vi "LCR_Main.vi"() -> ()   [LabVIEW 2021]
uses:
  Sources/Plotting-Axis.ctl
  GEN_States.ctl
  Sources/Config_Cluster.ctl
  Sources/Mode_Enum.ctl
  Sources/Data_Cluster.ctl
  Sources/Measurement_Cluster.ctl
  1375486a-d526-4950-a4e9-ede105372d37.vi
  <vilib>/Utility/config.llb/NI_LVConfig.lvlib
panel:
  in  "Control Tab":enum32{"LCR Operation", "Configs"}(tab)
  out "Magnetic Field":dbl
  out "Temperature":dbl
  in  "RefreshM_Button":bool
  in  "Operation Mode":enum32{"Item 0", "Item 1", "Radio Selection 3"}(radio)
  out "Time Stamp":timestamp format="%<%H:%M:%S>T"
  out "Secondary":dbl format="%#_6p"
  out "Primary":dbl format="%#_6p"
  in  "SaveProfile_Button":bool
  in  "Send_Button":bool
  in  "LoadProfile_Button":bool
  in  "Measurement Profile":path
  in  "Tab Control":T1(tab)
  in  "Auto Range (T: Enable)":bool=TRUE
  in  "Circuit Type (2: Auto)":u16(ring)=2 items=["Series", "Parallel", "Auto"]
  in  "Operation Mode (0: Auto)":u16(ring) items=["Auto", "L+Q", "L+R", "C+D", "C+R", "R+Q", "Z+Theta", "Y+Theta", "R+X", "G+B", "N+Theta", "M"]
  in  "Manual Range (1:Range 1 and 25 Ohms)":u8(ring)=1 items=["Range 1 and 25 Ohms"=1, "Range 2 and 25 Ohms"=2, "Range 3 and 400 Ohms"=3, "Range 4 and 6.4 kOhms"=4, "Range 5 and 100kOhms"=5, "Range 6 and 100kOhms"=6]
  in  "Bias Source (OFF)":u8(ring) items=["Off", "Internal", "External"]
  in  "Bias Level (0)":dbl
  in  "Bias Type (Voltage)":u8(ring) items=["Voltage", "Current"]
  in  "Averaging (0: Off)":u16(ring) items=["Off", "Normal", "Averaging"]
  in  "Averaging Number (2)":i32=2 min=2 max=99
  in  "Rate (0: Fast)":u16(ring) items=["Fast", "Medium", "Slow"]
  in  "Time (100ms)":i32=100 min=1 max=999
  in  "Frequency (1kHz)":dbl=1000.0 min=20.0 max=200000.0
  in  "Measuring Voltage (1V)":dbl=1.0 min=0.05 max=1.5 step=0.01
  in  "Trigger Mode (0: Continuous)":u16(ring) items=["Continuous", "Manual", "External"]
  in  "Logfile Prefix":string
  in  "Logging Path":path
  in  "Measure rate (1/s)":i32
  in  "SaveConfig_Button":bool
  in  "Default Measurement Profile":path
  in  "Retry_Button":bool
  in  "Restart on Load":bool
  in  "Config Path (Blank is default)":path
  in  "LCR VISA COM":refnum<visa-resource-name>
  in  "Max Elements":i32=5000
  in  "Global Temp VAR":refnum<k21>
  in  "Global Mag VAR":refnum<k21>
  in  "Display Tab":enum32{"Program Monitor", "Test Plot"}(tab)
  out "Status":string
  out "B Lag":dbl
  out "T Lag":dbl
  out "Test Graph":cluster{"X":dbl, "Y":dbl}[](graph)
  in  "Y-Axis":T2
  in  "X-Axis":T2
  in  "Exit_Button":bool
  # "R&S HM8118 Settings"
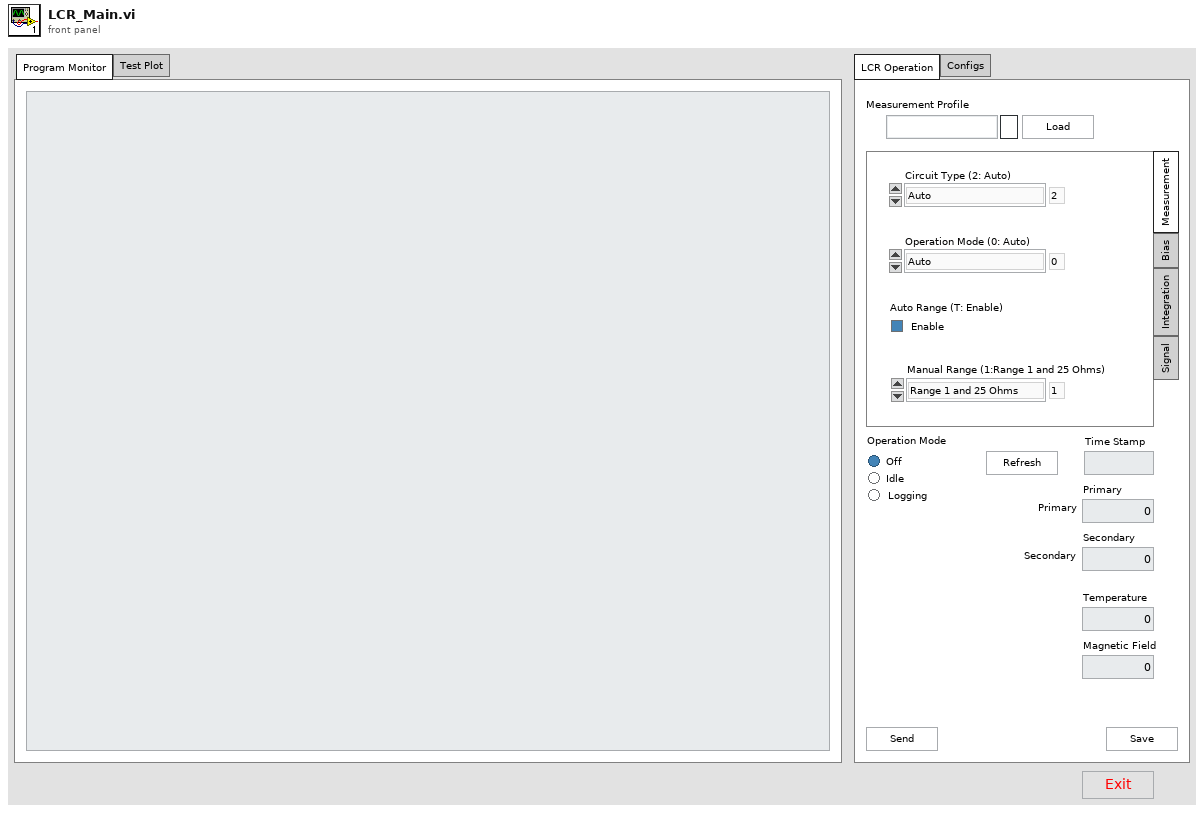
[diagram p1: front panel]
types:
  T1 = enum32{"Measurement", "Bias", "Integration", "Signal"}
  T2 = typedef "Plotting-Axis.ctl" = enum16{"Time", "Temperature", "MagneticField", "Primary", "Secondary"}
  T3 = typedef "GEN_States.ctl" = enum16{"UpdatePlots", "RefreshMUnits", "ChangeOperation", "Read/WriteAll", "RetryComs", "SendProfile", "InitGUI", "RefreshGUI", "ComsFail", "LoadProfile", "SaveProfile", "SaveConfig", "Idle", "ProgInit"}
  T4 = typedef "Data_Cluster.ctl" = cluster{"Value":dbl, "GUI Data Cluster":cluster{"Bias":cluster{"Bias Type (Voltage) 2":refnum<vi>, "Bias Level (0) 2":refnum<vi>, "Bias Source (OFF) 2":refnum<vi>}, "Measurement":cluster{"Auto Range (T: Enable) 2":refnum<vi>, "Manual Range (1:Range 1 and 25 Ohms) 2":refnum<vi>, "Operation Mode (0: Auto) 2":refnum<vi>, "Circuit Type (2: Auto) 2":refnum<vi>}, "Integration":cluster{"Rate (0: Fast) 2":refnum<vi>, "Time (100ms) 2":refnum<vi>, "Averaging (0: Off) 2":refnum<vi>, "Averaging Number (2) 2":refnum<vi>}, "Signal":cluster{"Trigger Mode (0: Continuous) 2":refnum<vi>, "Frequency (1kHz) 2":refnum<vi>, "Measuring Voltage (1V) 2":refnum<vi>}}, "Timing":cluster{"Last Operation":dbl}, "Measurements":T5[]}
  T5 = typedef "Measurement_Cluster.ctl" = cluster{"Time Stamp":timestamp, "Primary":dbl, "Secondary":dbl, "Temperature":dbl, "MagneticField":dbl}
  T6 = typedef "Config_Cluster.ctl" = cluster{"General":cluster{"Config.ini":path, "Default Logging Path":path}, "Hardware":cluster{"LCR VISA COM":refnum<visa-resource-name>, "Measure Rate (1/s)":i32, "Reset on Load?":bool, "Measure Profile":path, "Global T VAR":refnum<k21>, "Global B VAR":refnum<k21>}, "HM8118 Current Profile":cluster{"Bias Profile":cluster{" Bias Source (OFF)":u8, " Bias Type (Voltage)":u8, "Bias Level (0)":dbl}, "Measurement Profile":cluster{"Operation Mode (0: Auto)":u16, "Circuit Type (2: Auto)":u16, "Manual Range (1:Range 1 and 25 Ohms)":u8, "Auto Range (T: Enable)":bool}, "Signal Profile":cluster{"Frequency (1kHz)":dbl, "Measuring Voltage (1V)":dbl}, "Integration Profile":cluster{"Averaging (0: Off)":u16, "Averaging Number (2)":i32, "Time (100ms)":i32, "Rate (0: Fast)":u16}, "Trigger Profile":cluster{"Trigger Mode (0: Continuous)":u16}}, "HM8118 New Profile":cluster{"Bias Profile":cluster{" Bias Source (OFF)":u8, " Bias Type (Voltage)":u8, "Bias Level (0)":dbl}, "Measurement Profile":cluster{"Operation Mode (0: Auto)":u16, "Circuit Type (2: Auto)":u16, "Manual Range (1:Range 1 and 25 Ohms)":u8, "Auto Range (T: Enable)":bool}, "Signal Profile":cluster{"Frequency (1kHz)":dbl, "Measuring Voltage (1V)":dbl}, "Integration Profile":cluster{"Averaging (0: Off)":u16, "Averaging Number (2)":i32, "Time (100ms)":i32, "Rate (0: Fast)":u16}, "Trigger Profile":cluster{"Trigger Mode (0: Continuous)":u16}}, "Operation":cluster{"Operation Mode":T7, "Status":string}}
  T7 = typedef "Mode_Enum.ctl" = enum16{"Logging", "Idle-Off", "Idle"}
  T8 = enum8{"Enabled", "Disabled", "Disabled and Grayed Out"}
  T9 = typedef "NI_LVConfig.lvlib/Config Data RefNum.ctl" = refnum<k1>
  T10 = cluster{"Logging Path":path, "LCR VISA COM":refnum<visa-resource-name>, "Restart on Load":bool, "Default Measurement Profile":path, "Measure rate (1/s)":i32}
  T11 = cluster{"Primary Measurement":dbl, "Secondary Measurement":dbl, "T Var":dbl, "B Var":dbl}
  T12 = typedef "UnitEnum.ctl" = enum16{"L", "R", "C", "Z", "X", "Q", "Theta", "Y", "N", "M", "G", "B", "D"}
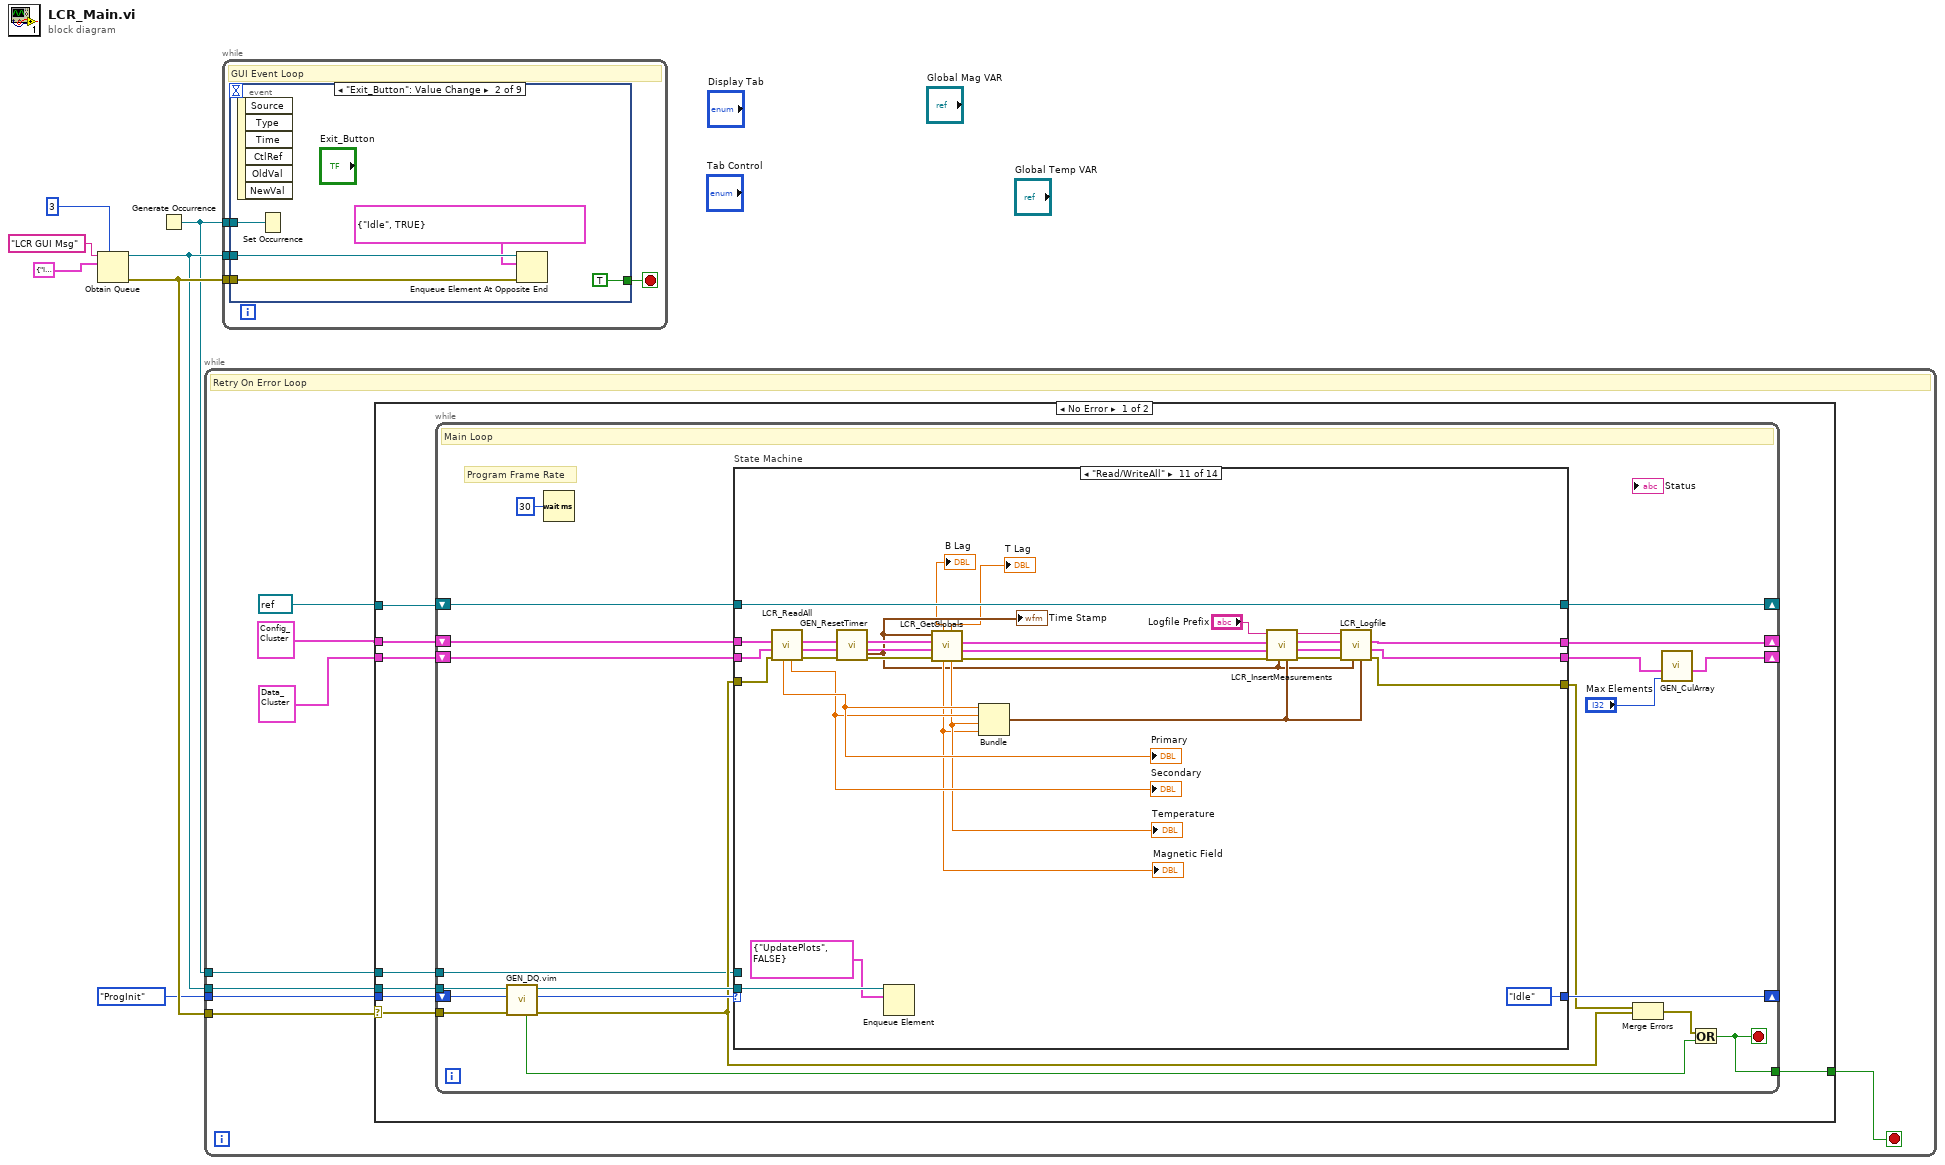
[diagram p0: block diagram]
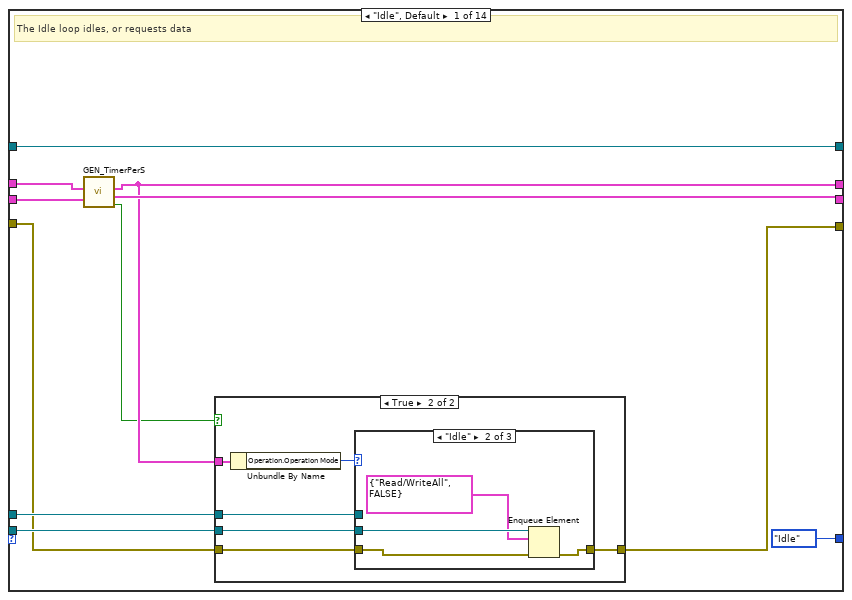
[diagram p2: hidden frame]
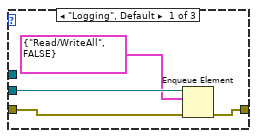
[diagram p4: hidden frame]
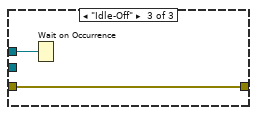
[diagram p5: hidden frame]
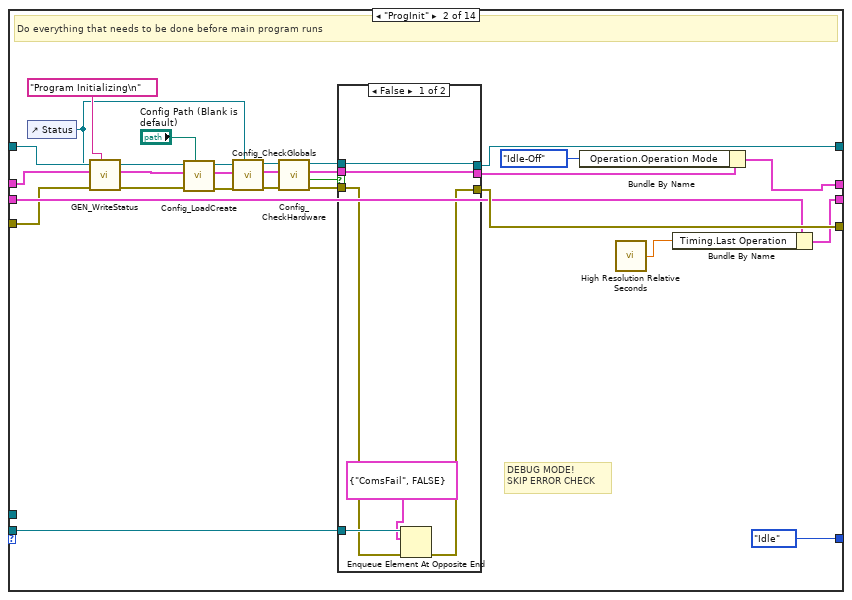
[diagram p6: hidden frame]
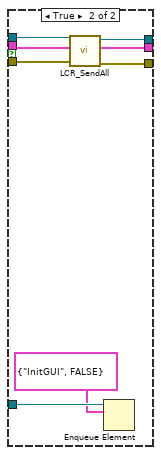
[diagram p7: hidden frame]
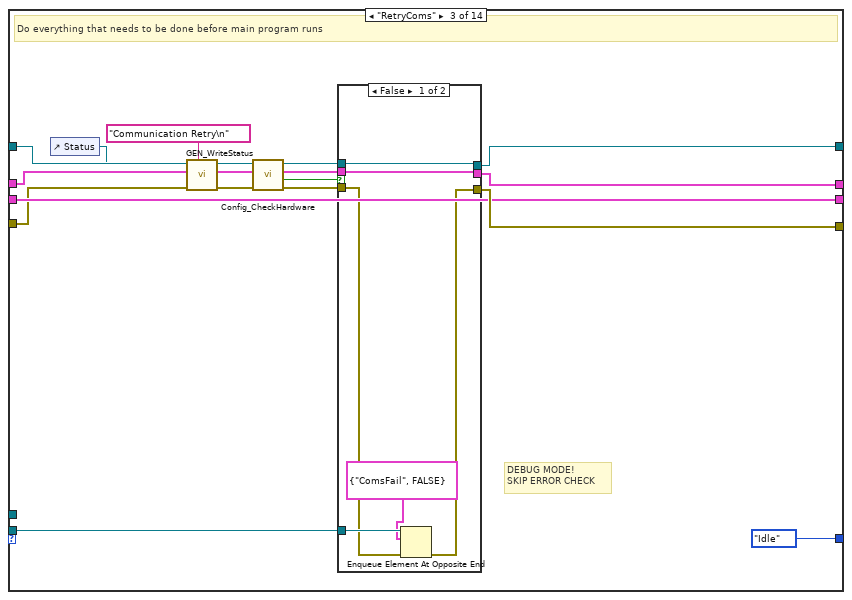
[diagram p8: hidden frame]
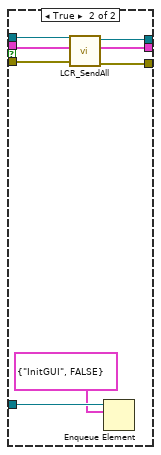
[diagram p9: hidden frame]
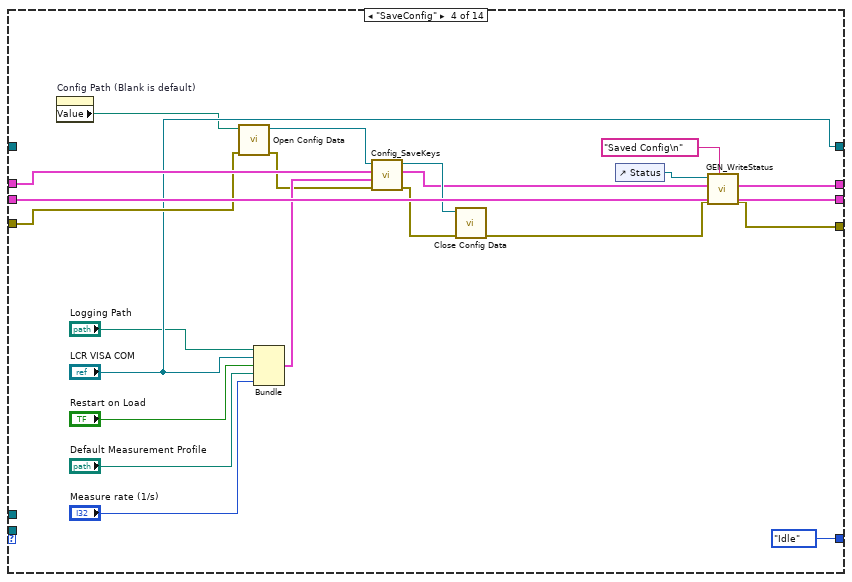
[diagram p10: hidden frame]
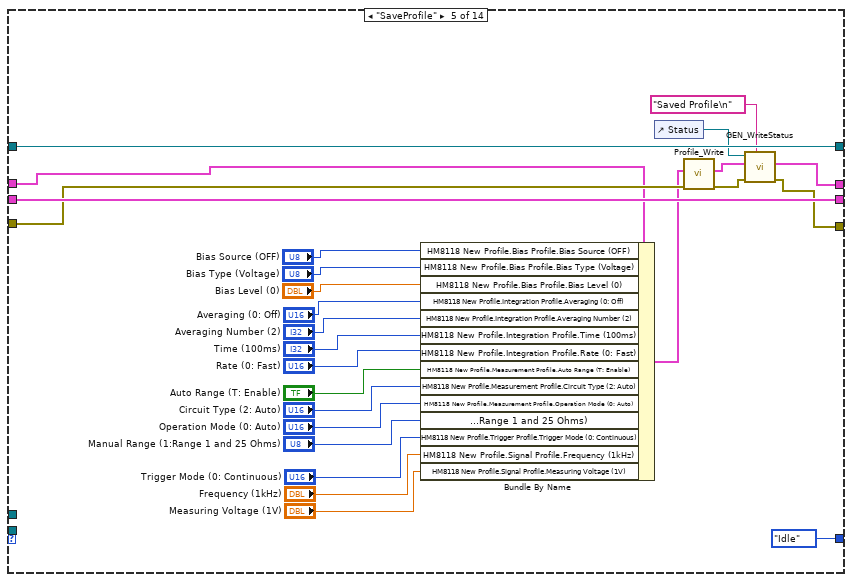
[diagram p11: hidden frame]
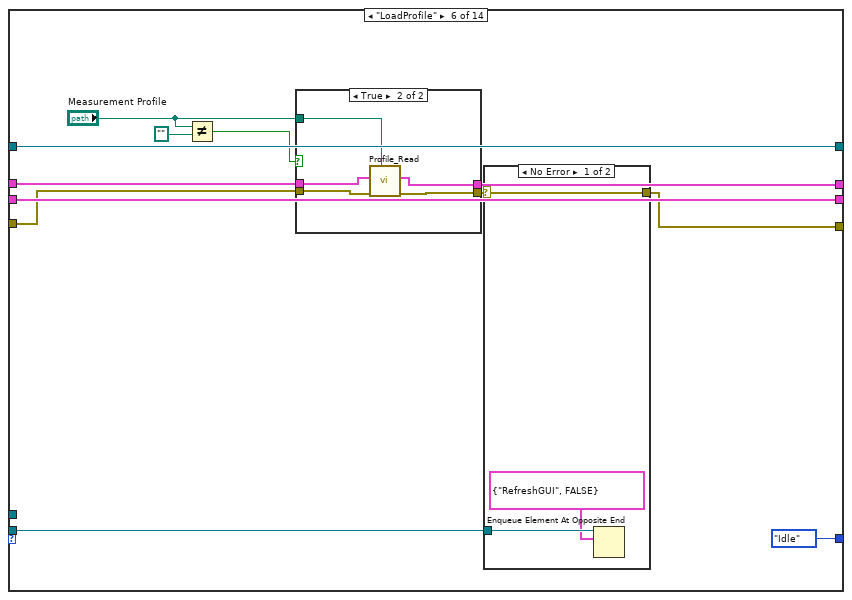
[diagram p12: hidden frame]
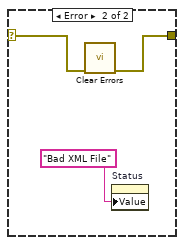
[diagram p13: hidden frame]
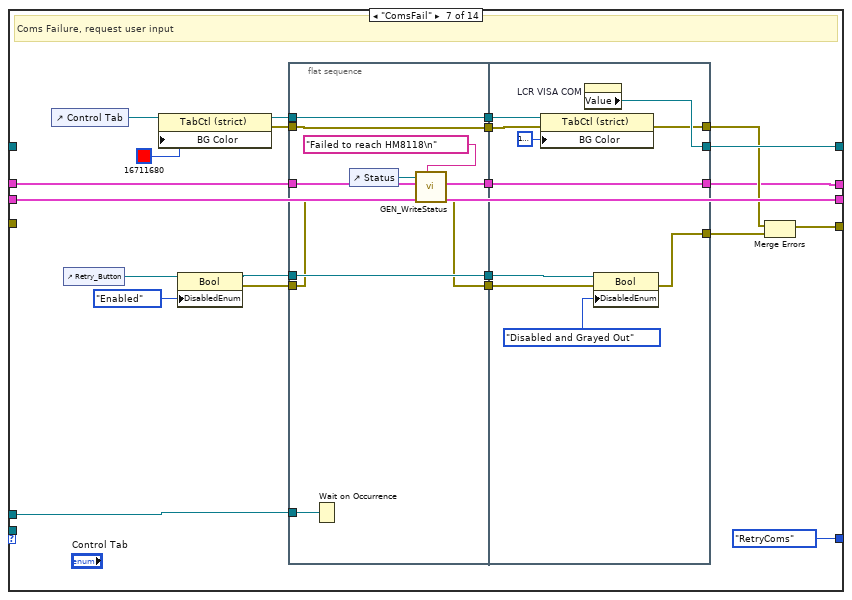
[diagram p15: hidden frame]
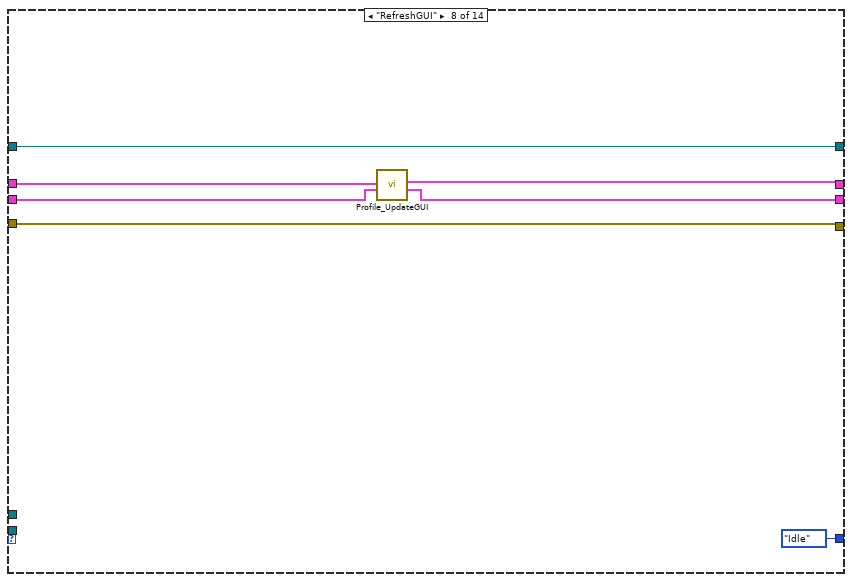
[diagram p16: hidden frame]
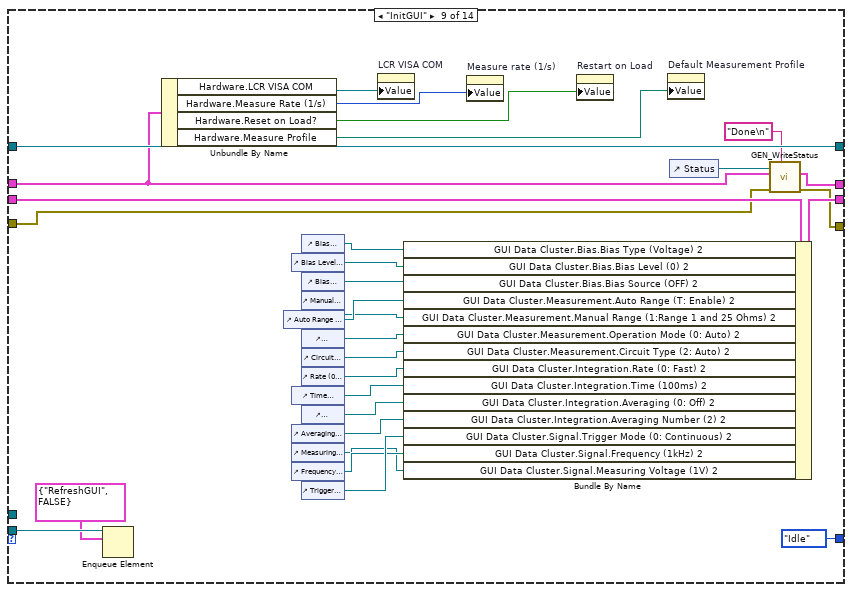
[diagram p17: hidden frame]
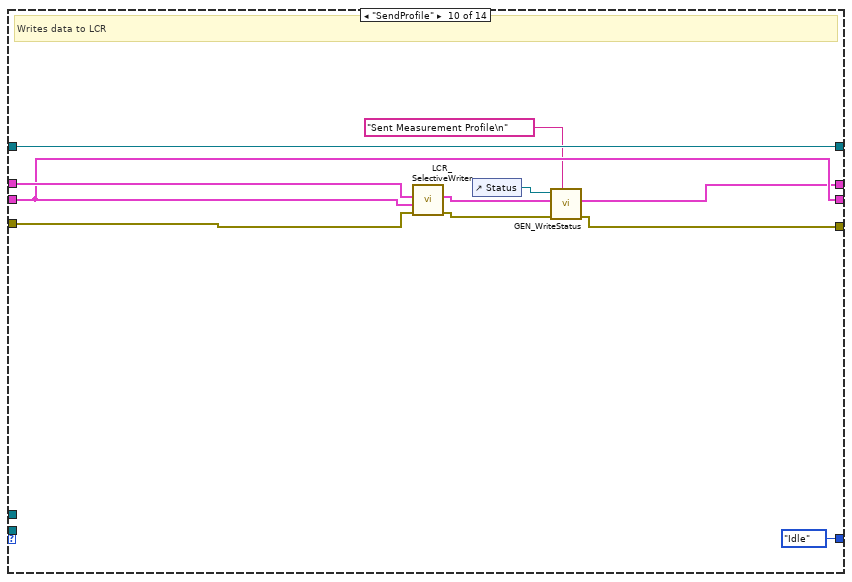
[diagram p18: hidden frame]
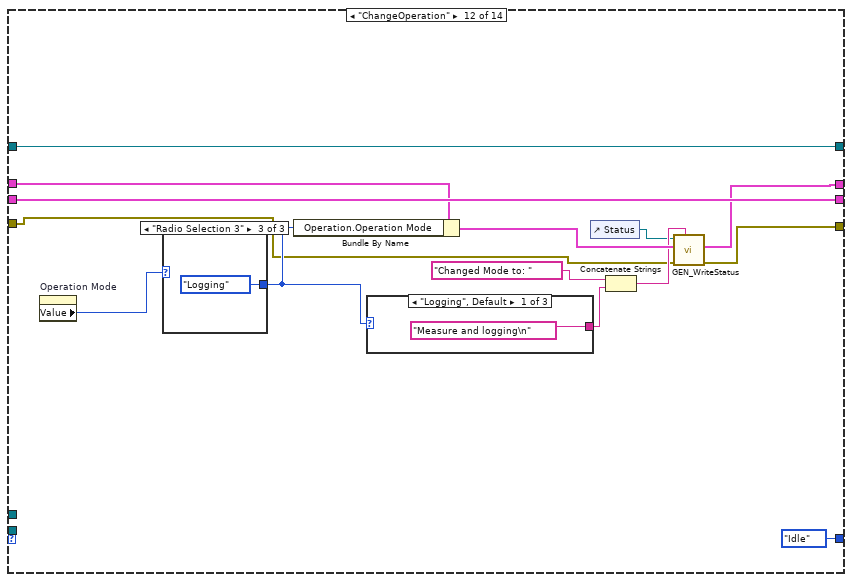
[diagram p19: hidden frame]
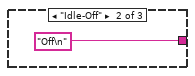
[diagram p20: hidden frame]
diagram:
  n1 = Obtain Queue(max queue size (-1, unlimited)=3, name (unnamed)="LCR GUI Msg", element data type=cluster{T3, bool} {enum."Idle", TRUE}) -> (queue out=w3:refnum<queue>, error out=w4:errorcluster)  [unwired: 2 in, 1 out]
  n2 = Generate Occurrence() -> (w1:refnum<k4>)
  n3 = while {
    tunnel: w4 -> [w15]
    tunnel: w3 -> [w14]
    tunnel: GEN_States."ProgInit" ("State") -> [w13]
    tunnel: w1 -> [w8]
    stop <- w12 stop-if-true
    # "Retry On Error Loop"
    n4 = case shown="No Error" w15 {
      selector: w15 -> [w23 _]
      tunnel: w14 -> [w22 _]
      tunnel: w13 -> [w21 _]
      tunnel: [w20 TRUE] -> w12
      tunnel: refnum<visa-resource-name> refnum ("LCR VISA COM") -> [w19 _]
      tunnel: T6 {"General"={"Config.ini"=path "", "Default Logging Path"=path ""}, "Hardware"={"LCR VISA COM"="", "Measure Rate (1/s)"=0, "Reset on Load?"=FALSE, "Measure Profile"=path "", "Global T VAR"="", "Global B VAR"=""}, "HM8118 Current Profile"={"Bias Profile"={" Bias Source (OFF)"=0, " Bias Type (Voltage)"=0, "Bias Level (0)"=0.0}, "Measurement Profile"={"Operation Mode (0: Auto)"=0, "Circuit Type (2: Auto)"=0, "Manual Range (1:Range 1 and 25 Ohms)"=0, "Auto Range (T: Enable)"=FALSE}, "Signal Profile"={"Frequency (1kHz)"=0.0, "Measuring Voltage (1V)"=0.0}, "Integration Profile"={"Averaging (0: Off)"=0, "Averaging Number (2)"=0, "Time (100ms)"=0, "Rate (0: Fast)"=0}, "Trigger Profile"={"Trigger Mode (0: Continuous)"=0}}, "HM8118 New Profile"={"Bias Profile"={" Bias Source (OFF)"=0, " Bias Type (Voltage)"=0, "Bias Level (0)"=0.0}, "Measurement Profile"={"Operation Mode (0: Auto)"=0, "Circuit Type (2: Auto)"=0, "Manual Range (1:Range 1 and 25 Ohms)"=0, "Auto Range (T: Enable)"=FALSE}, "Signal Profile"={"Frequency (1kHz)"=0.0, "Measuring Voltage (1V)"=0.0}, "Integration Profile"={"Averaging (0: Off)"=0, "Averaging Number (2)"=0, "Time (100ms)"=0, "Rate (0: Fast)"=0}, "Trigger Profile"={"Trigger Mode (0: Continuous)"=0}}, "Operation"={"Operation Mode"=enum."Logging", "Status"=""}} -> [w18 _]
      tunnel: T4 {"Value"=0.0, "GUI Data Cluster"={"Bias"={"Bias Type (Voltage) 2"=refnum, "Bias Level (0) 2"=refnum, "Bias Source (OFF) 2"=refnum}, "Measurement"={"Auto Range (T: Enable) 2"=refnum, "Manual Range (1:Range 1 and 25 Ohms) 2"=refnum, "Operation Mode (0: Auto) 2"=refnum, "Circuit Type (2: Auto) 2"=refnum}, "Integration"={"Rate (0: Fast) 2"=refnum, "Time (100ms) 2"=refnum, "Averaging (0: Off) 2"=refnum, "Averaging Number (2) 2"=refnum}, "Signal"={"Trigger Mode (0: Continuous) 2"=refnum, "Frequency (1kHz) 2"=refnum, "Measuring Voltage (1V) 2"=refnum}}, "Timing"={"Last Operation"=0.0}, "Measurements"=[]} -> [w17 _]
      tunnel: w8 -> [w16 _]
      frame No Error {
        n5 = while {
          tunnel: w23 -> [w43]
          tunnel: w22 -> [w42]
          shift-right: [w35] -> _
          shift-left: w21 -> [w41]
          tunnel: [w37] -> w20
          shift-right: [w34] -> _
          shift-left: w19 -> [w36]
          shift-right: [w31] -> _
          shift-left: w18 -> [w32]
          shift-right: [w25] -> _
          shift-left: w17 -> [w30]
          tunnel: w16 -> [w27]
          stop <- w37 stop-if-true
          # "Program Frame Rate"
          # "Main Loop"
          n6 = call "GEN_DQ.vim"("error in (no error)"=w43, "Variant"=w41, "queue In"=w42) -> ("error out"=w29:errorcluster, "Variant Out"=w40:T3, "queue out"=w33:refnum<queue>, "Exit?"=w38:bool)  [unwired: 5 in]
          n7 = Wait (ms)(milliseconds to wait=u32 30) -> ()  [unwired: 1 out]
          n8 = case "State Machine" shown="\"Read/WriteAll\"" w40 {
            tunnel: w36 -> [w55 w98 w130 _ w192 w204 _ w265 w296 w307 w338 w352 w368 w379]
            tunnel: [GEN_States."Idle" ("State") GEN_States."Idle" ("State") GEN_States."Idle" ("State") GEN_States."Idle" ("State") GEN_States."Idle" ("State") GEN_States."Idle" ("State") GEN_States."RetryComs" ("State") GEN_States."Idle" ("State") GEN_States."Idle" ("State") GEN_States."Idle" ("State") GEN_States."Idle" ("State") GEN_States."Idle" ("State") GEN_States."Idle" ("State") GEN_States."Idle" ("State")] -> w35
            tunnel: [w55 w92 w123 "LCR VISA COM" w192 w204 w232 w265 w296 w307 w338 w352 w368 w379] -> w34
            tunnel: w33 -> [w52 w91 w122 _ _ w193 _ _ w292 _ w331 _ _ _]
            tunnel: w32 -> [w49 w83 w120 w160 w188 w200 w220 w260 w272 w306 w337 w350 w369 w378]
            tunnel: [w46 w84 w124 w150 w171 w199 w219 w262 w271 w301 w332 w346 w366 w378] -> w31
            tunnel: w30 -> [w48 w90 w121 w166 w191 w203 w234 w263 w295 w304 w326 w351 w367 w374]
            tunnel: [w47 w89 w121 w166 w191 w203 w234 w261 w294 w304 w322 w351 w367 w373] -> w26
            tunnel: w29 -> [w51 w81 w117 w159 w189 w201 _ w264 w269 w305 w336 w341 w365 w372]
            tunnel: [w50 w93 w125 w146 w168 w194 w223 w264 w268 w298 w333 w340 w360 w372] -> w28
            tunnel: w27 -> [w53 _ _ _ _ _ w233 _ _ _ _ _ _ _]
            frame "Idle", Default {
              # "The Idle loop idles, or requests data"
              n9 = call "GEN_TimerPerS.vi"("Data_In"=w48, "Config_In"=w49) -> ("Time"=w45:bool, "Data_In 2"=w47:T4, "Config_In 2"=w46:T6)  [unwired: 7 in]
              n10 = case shown="True" w45 {
                tunnel: w53 -> [_ w61]
                tunnel: w52 -> [_ w60]
                tunnel: w51 -> [w56 w59]
                tunnel: [w56 w58] -> w50
                tunnel: w46 -> [_ w57]
                frame False {
                }
                frame True {
                  n11 = Unbundle By Name(w57) -> ("Operation.Operation Mode"=w62:T7)
                  n12 = case shown="\"Idle\"" w62 {
                    tunnel: w61 -> [_ _ w72]
                    tunnel: w60 -> [w66 w70 _]
                    tunnel: w59 -> [w65 w69 w71]
                    tunnel: [w63 w67 w71] -> w58
                    frame "Logging", Default {
                      n13 = Enqueue Element(queue=w66, element=cluster{T3, bool} {enum."Read/WriteAll", FALSE}, error in (no error)=w65) -> (error out=w63:errorcluster)  [unwired: 1 in, 2 out]
                    }
                    frame "Idle" {
                      n14 = Enqueue Element(queue=w70, element=cluster{T3, bool} {enum."Read/WriteAll", FALSE}, error in (no error)=w69) -> (error out=w67:errorcluster)  [unwired: 1 in, 2 out]
                    }
                    frame "Idle-Off" {
                      n15 = Wait on Occurrence(2:w72) -> ()  [unwired: 2 in, 1 out]
                    }
                  }
                }
              }
            }
            frame "ProgInit" {
              # "DEBUG MODE!\nSKIP ERROR CHECK"
              # "Do everything that needs to be done before main program runs"
              n16 = control-ref of="Status"() -> (w73:refnum<vi>)
              n17 = call "GEN_WriteStatus.vi"("Input String"="Program Initializing\n" ("Status"), "error in (no error)"=w81, "Config_Cluster"=w83, "Status Ref"=w73) -> ("error out"=w80:errorcluster, "Config_Cluster Out"=w82:T6)  [unwired: 6 in]
              n18 = call "Config_LoadCreate.vi"("Config In"="Config Path (Blank is default)", "error In"=w80, "Configuration Cluster"=w82, "LCR VISA COM"=w98) -> ("error out"=w75:errorcluster, "Configuration Cluster Out"=w76:T6, "LCR VISA COM Out"=w79:refnum<visa-resource-name>)  [unwired: 5 in]
              n19 = call "Config_CheckGlobals.vi"("Status Ref"=w73, "error in (no error)"=w75, "Config Cluster"=w76, "VISA resource name"=w79) -> ("error out"=w74:errorcluster, "Config Cluster Out"=w77:T6, "VISA resource name out"=w78:refnum<visa-resource-name>)  [unwired: 5 in]
              n20 = call "Config_CheckHardware.vi"("error in (no error)"=w74, "Config Cluster"=w77, "VISA resource name"=w78) -> ("error out"=w96:errorcluster, "Connected?"=w97:bool, "Config Cluster Out"=w95:T6, "VISA resource name out"=w94:refnum<visa-resource-name>)  [unwired: 5 in]
              n21 = case shown="False" w97 {
                tunnel: w96 -> [w102 w112]
                tunnel: w95 -> [w105 w113]
                tunnel: w94 -> [w106 w114]
                tunnel: [w106 w111] -> w92
                tunnel: [w105 w110] -> w87
                tunnel: [w101 w109] -> w93
                tunnel: w91 -> [w104 w108]
                frame False {
                  n22 = Enqueue Element At Opposite End(queue=w104, element=cluster{T3, bool} {enum."ComsFail", FALSE}, error in (no error)=w102) -> (error out=w101:errorcluster)  [unwired: 1 in, 2 out]
                }
                frame True {
                  n23 = call "LCR_SendAll.vi"("error in (no error)"=w112, "Configuration Cluster"=w113, "VISA resource name"=w114) -> ("error out"=w109:errorcluster, "Configuration Cluster Out"=w110:T6, "VISA resource name out"=w111:refnum<visa-resource-name>)  [unwired: 6 in]
                  n24 = Enqueue Element(queue=w108, element=cluster{T3, bool} {enum."InitGUI", FALSE}) -> ()  [unwired: 2 in, 3 out]
                }
              }
              n25 = Bundle By Name(cluster=w87, "Operation.Operation Mode"=Mode_Enum."Idle-Off") -> (w84:T6)
              n26 = call <vilib>:"High Resolution Relative Seconds.vi"() -> ("relative seconds"=w88:dbl)
              n27 = Bundle By Name(cluster=w90, "Timing.Last Operation"=w88) -> (w89:T4)
            }
            frame "RetryComs" {
              # "DEBUG MODE!\nSKIP ERROR CHECK"
              # "Do everything that needs to be done before main program runs"
              n28 = control-ref of="Status"() -> (w115:refnum<vi>)
              n29 = call "GEN_WriteStatus.vi"("Input String"="Communication Retry\n", "error in (no error)"=w117, "Config_Cluster"=w120, "Status Ref"=w115) -> ("error out"=w116:errorcluster, "Config_Cluster Out"=w119:T6)  [unwired: 6 in]
              n30 = call "Config_CheckHardware.vi"("error in (no error)"=w116, "Config Cluster"=w119, "VISA resource name"=w130) -> ("error out"=w128:errorcluster, "Connected?"=w129:bool, "Config Cluster Out"=w127:T6, "VISA resource name out"=w126:refnum<visa-resource-name>)  [unwired: 5 in]
              n31 = case shown="False" w129 {
                tunnel: w128 -> [w133 w143]
                tunnel: w127 -> [w136 w144]
                tunnel: w126 -> [w137 w145]
                tunnel: [w137 w142] -> w123
                tunnel: [w136 w141] -> w124
                tunnel: [w132 w140] -> w125
                tunnel: w122 -> [w135 w139]
                frame False {
                  n32 = Enqueue Element At Opposite End(queue=w135, element=cluster{T3, bool} {enum."ComsFail", FALSE}, error in (no error)=w133) -> (error out=w132:errorcluster)  [unwired: 1 in, 2 out]
                }
                frame True {
                  n33 = call "LCR_SendAll.vi"("error in (no error)"=w143, "Configuration Cluster"=w144, "VISA resource name"=w145) -> ("error out"=w140:errorcluster, "Configuration Cluster Out"=w141:T6, "VISA resource name out"=w142:refnum<visa-resource-name>)  [unwired: 6 in]
                  n34 = Enqueue Element(queue=w139, element=cluster{T3, bool} {enum."InitGUI", FALSE}) -> ()  [unwired: 2 in, 3 out]
                }
              }
            }
            frame "SaveConfig" {
              n35 = property on="Config Path (Blank is default)" class="Path"() -> ("Value"=w153:path)  [unwired: 2 in, 2 out]
              n36 = call <vilib>:"Open Config Data.vi"("error in (no error)"=w159, "configuration file path"=w153) -> ("error out"=w158:errorcluster, "refnum"=w157:T9)  [unwired: 7 in, 1 out]
              n37 = Bundle("Logging Path"="Logging Path", "LCR VISA COM"="LCR VISA COM", "Restart on Load"="Restart on Load", "Default Measurement Profile"="Default Measurement Profile", "Measure rate (1/s)"="Measure rate (1/s)") -> (w161:T10)  [unwired: 1 in]
              n38 = call "Config_SaveKeys.vi"("error in (no error)"=w158, "Settings IN"=w161, "Configuration Cluster"=w160, "Config In"=w157) -> ("error out"=w155:errorcluster, "output cluster"=w151:T6, "refnum out"=w156:T9)  [unwired: 5 in]
              n39 = call <vilib>:"Close Config Data.vi"("error in (no error)"=w155, "refnum"=w156) -> ("error out"=w147:errorcluster)  [unwired: 8 in, 1 out]
              n40 = control-ref of="Status"() -> (w148:refnum<vi>)
              n41 = call "GEN_WriteStatus.vi"("Input String"="Saved Config\n", "error in (no error)"=w147, "Config_Cluster"=w151, "Status Ref"=w148) -> ("error out"=w146:errorcluster, "Config_Cluster Out"=w150:T6)  [unwired: 6 in]
            }
            frame "SaveProfile" {
              n42 = Bundle By Name(cluster=w188, "HM8118 New Profile.Bias Profile.Bias Source (OFF)"="Bias Source (OFF)", "HM8118 New Profile.Bias Profile.Bias Type (Voltage)"="Bias Type (Voltage)", "HM8118 New Profile.Bias Profile.Bias Level (0)"="Bias Level (0)", "HM8118 New Profile.Integration Profile.Averaging (0: Off)"="Averaging (0: Off)", "HM8118 New Profile.Integration Profile.Averaging Number (2)"="Averaging Number (2)", "HM8118 New Profile.Integration Profile.Time (100ms)"="Time (100ms)", "HM8118 New Profile.Integration Profile.Rate (0: Fast)"="Rate (0: Fast)", "HM8118 New Profile.Measurement Profile.Auto Range (T: Enable)"="Auto Range (T: Enable)", "HM8118 New Profile.Measurement Profile.Circuit Type (2: Auto)"="Circuit Type (2: Auto)", "HM8118 New Profile.Measurement Profile.Operation Mode (0: Auto)"="Operation Mode (0: Auto)", "HM8118 New Profile.Measurement Profile.Manual Range (1:Range 1 and 25 Ohms)"="Manual Range (1:Range 1 and 25 Ohms)", "HM8118 New Profile.Trigger Profile.Trigger Mode (0: Continuous)"="Trigger Mode (0: Continuous)", "HM8118 New Profile.Signal Profile.Frequency (1kHz)"="Frequency (1kHz)", "HM8118 New Profile.Signal Profile.Measuring Voltage (1V)"="Measuring Voltage (1V)") -> (w187:T6)
              n43 = control-ref of="Status"() -> (w167:refnum<vi>)
              n44 = call "Profile_Write.vi"("error in"=w189, "Configuration Cluster"=w187) -> ("error out"=w169:errorcluster, "Configuration Cluster Out"=w172:T6)  [unwired: 8 in]
              n45 = call "GEN_WriteStatus.vi"("Input String"="Saved Profile\n", "error in (no error)"=w169, "Config_Cluster"=w172, "Status Ref"=w167) -> ("error out"=w168:errorcluster, "Config_Cluster Out"=w171:T6)  [unwired: 6 in]
            }
            frame "LoadProfile" {
              n46 = Not Equal?(x="Measurement Profile", y=path "") -> (x != y?=w196:bool)
              n47 = case shown="True" w196 {
                tunnel: w201 -> [w211 w217]
                tunnel: w200 -> [w212 w216]
                tunnel: "Measurement Profile" -> [_ w215]
                tunnel: [w211 w214] -> w195
                tunnel: [w212 w213] -> w199
                frame False {
                }
                frame True {
                  n48 = call "Profile_Read.vi"("Measurement Profile"=w215, "error in (no error)"=w217, "Configuration Cluster"=w216) -> ("error out"=w214:errorcluster, "Configuration Cluster Out"=w213:T6)  [unwired: 7 in]
                }
              }
              n49 = case shown="No Error" w195 {
                selector: w195 -> [w207 w210]
                tunnel: [w207 w209] -> w194
                tunnel: w193 -> [w206 _]
                frame No Error {
                  n50 = Enqueue Element At Opposite End(queue=w206, element=cluster{T3, bool} {enum."RefreshGUI", FALSE}) -> ()  [unwired: 2 in, 3 out]
                }
                frame Error {
                  n51 = call <vilib>:"Clear Errors.vi"("error in (no error)"=w210) -> ("error out"=w209:errorcluster)  [unwired: 5 in, 1 out]
                  n52 = property on="Status" class="Str"("Value"="Bad XML File" ("Status")) -> ()  [unwired: 2 in, 2 out]
                }
              }
            }
            frame "ComsFail" {
              # "Coms Failure, request user input"
              n53 = control-ref of="Control Tab"() -> (w239:refnum<vi>)
              n54 = control-ref of="Retry_Button"() -> (w238:refnum<vi>)
              n55 = property on="Property Node" class="TabCtl (strict)"(reference=w239, "BG Color"=u32 16711680 ("Colors:BG Color")) -> (reference out=w230:refnum<vi>, error out=w229:errorcluster)  [unwired: 1 in]
              n56 = property class="Bool"(reference=w238, "DisabledEnum"=T8."Enabled" ("Disabled")) -> (reference out=w226:refnum<vi>, error out=w225:errorcluster)  [unwired: 1 in]
              n57 = flat-sequence {
                tunnel: w233 -> [w249]
                tunnel: [w248] -> w231
                tunnel: w230 -> [w248]
                tunnel: w229 -> [w247]
                tunnel: [w247] -> w228
                tunnel: [w246] -> w227
                tunnel: w226 -> [w246]
                tunnel: w225 -> [w242]
                tunnel: [w241] -> w224
                tunnel: w220 -> [w245]
                tunnel: [w244] -> w218
                tunnel: [w259] -> w232
                tunnel: w231 -> [w258]
                tunnel: w228 -> [w257]
                tunnel: w227 -> [w256]
                tunnel: w224 -> [w255]
                tunnel: [w253] -> w222
                tunnel: [w252] -> w221
                tunnel: [w250] -> w219
                tunnel: w218 -> [w250]
                frame #0 {
                  n58 = Wait on Occurrence(2:w249) -> ()  [unwired: 2 in, 1 out]
                  n59 = control-ref of="Status"() -> (w240:refnum<vi>)
                  n60 = call "GEN_WriteStatus.vi"("Input String"="Failed to reach HM8118\n", "error in (no error)"=w242, "Config_Cluster"=w245, "Status Ref"=w240) -> ("error out"=w241:errorcluster, "Config_Cluster Out"=w244:T6)  [unwired: 6 in]
                }
                frame #1 {
                  n61 = property class="TabCtl (strict)"(reference=w258, error in=w257, "BG Color"=u32 16777226 ("Colors:BG Color")) -> (error out=w253:errorcluster)  [unwired: 1 out]
                  n62 = property on="LCR VISA COM" class="VISAName"() -> ("Value"=w259:refnum<visa-resource-name>)  [unwired: 2 in, 2 out]
                  n63 = property class="Bool"(reference=w256, error in=w255, "DisabledEnum"=T8."Disabled and Grayed Out" ("Disabled")) -> (error out=w252:errorcluster)  [unwired: 1 out]
                }
              }
              n64 = Merge Errors(w222, w221) -> (w223:errorcluster)
            }
            frame "RefreshGUI" {
              n65 = call "Profile_UpdateGUI.vi"("Data Cluster"=w263, "Configuration Cluster"=w260) -> ("Data Cluster Out"=w261:T4, "Configuration Cluster Out"=w262:T6)  [unwired: 8 in]
            }
            frame "InitGUI" {
              n66 = Enqueue Element(queue=w292, element=cluster{T3, bool} {enum."RefreshGUI", FALSE}) -> ()  [unwired: 2 in, 3 out]
              n67 = Unbundle By Name(w272) -> ("Hardware.LCR VISA COM"=w276:refnum<visa-resource-name>, "Hardware.Measure Rate (1/s)"=w275:i32, "Hardware.Reset on Load?"=w274:bool, "Hardware.Measure Profile"=w273:path)
              n68 = control-ref of="Auto Range (T: Enable)"() -> (w287:refnum<vi>)
              n69 = control-ref of="Bias Level (0)"() -> (w289:refnum<vi>)
              n70 = control-ref of="Time (100ms)"() -> (w281:refnum<vi>)
              n71 = control-ref of="Averaging Number (2)"() -> (w280:refnum<vi>)
              n72 = control-ref of="Measuring Voltage (1V)"() -> (w277:refnum<vi>)
              n73 = control-ref of="Frequency (1kHz)"() -> (w278:refnum<vi>)
              n74 = control-ref of="Bias Type (Voltage)"() -> (w290:refnum<vi>)
              n75 = control-ref of="Bias Source (OFF)"() -> (w288:refnum<vi>)
              n76 = control-ref of="Manual Range (1:Range 1 and 25 Ohms)"() -> (w286:refnum<vi>)
              n77 = control-ref of="Operation Mode (0: Auto)"() -> (w285:refnum<vi>)
              n78 = control-ref of="Circuit Type (2: Auto)"() -> (w284:refnum<vi>)
              n79 = control-ref of="Rate (0: Fast)"() -> (w283:refnum<vi>)
              n80 = control-ref of="Averaging (0: Off)"() -> (w282:refnum<vi>)
              n81 = control-ref of="Trigger Mode (0: Continuous)"() -> (w279:refnum<vi>)
              n82 = property on="LCR VISA COM" class="VISAName"("Value"=w276) -> ()  [unwired: 2 in, 2 out]
              n83 = Bundle By Name(cluster=w295, "GUI Data Cluster.Bias.Bias Type (Voltage) 2"=w290, "GUI Data Cluster.Bias.Bias Level (0) 2"=w289, "GUI Data Cluster.Bias.Bias Source (OFF) 2"=w288, "GUI Data Cluster.Measurement.Auto Range (T: Enable) 2"=w287, "GUI Data Cluster.Measurement.Manual Range (1:Range 1 and 25 Ohms) 2"=w286, "GUI Data Cluster.Measurement.Operation Mode (0: Auto) 2"=w285, "GUI Data Cluster.Measurement.Circuit Type (2: Auto) 2"=w284, "GUI Data Cluster.Integration.Rate (0: Fast) 2"=w283, "GUI Data Cluster.Integration.Time (100ms) 2"=w281, "GUI Data Cluster.Integration.Averaging (0: Off) 2"=w282, "GUI Data Cluster.Integration.Averaging Number (2) 2"=w280, "GUI Data Cluster.Signal.Trigger Mode (0: Continuous) 2"=w279, "GUI Data Cluster.Signal.Frequency (1kHz) 2"=w278, "GUI Data Cluster.Signal.Measuring Voltage (1V) 2"=w277) -> (w294:T4)
              n84 = property on="Measure rate (1/s)" class="DigNum (strict)"("Value"=w275) -> ()  [unwired: 2 in, 2 out]
              n85 = property on="Restart on Load" class="Bool (strict)"("Value"=w274) -> ()  [unwired: 2 in, 2 out]
              n86 = property on="Default Measurement Profile" class="Path"("Value"=w273) -> ()  [unwired: 2 in, 2 out]
              n87 = control-ref of="Status"() -> (w267:refnum<vi>)
              n88 = call "GEN_WriteStatus.vi"("Input String"="Done\n", "error in (no error)"=w269, "Config_Cluster"=w272, "Status Ref"=w267) -> ("error out"=w268:errorcluster, "Config_Cluster Out"=w271:T6)  [unwired: 6 in]
            }
            frame "SendProfile" {
              # "Writes data to LCR"
              n89 = call "LCR_SelectiveWriter.vi"("error in (no error)"=w305, "Data Cluster"=w304, "Configuration Cluster"=w306) -> ("error out"=w299:errorcluster, "Configuration Cluster Out"=w302:T6)  [unwired: 7 in]
              n90 = control-ref of="Status"() -> (w297:refnum<vi>)
              n91 = call "GEN_WriteStatus.vi"("Input String"="Sent Measurement Profile\n", "error in (no error)"=w299, "Config_Cluster"=w302, "Status Ref"=w297) -> ("error out"=w298:errorcluster, "Config_Cluster Out"=w301:T6)  [unwired: 6 in]
            }
            frame "Read/WriteAll" {
              n92 = call "LCR_ReadAll.vi"("error in (no error)"=w336, "Data_In"=w326, "Configuration Cluster"=w337) -> ("error out"=w335:errorcluster, "Data_Out"=w325:T4, "Configuration Cluster 2"=w329:T6, "Secondary Measurement"=w320:dbl, "Primary Measurement"=w321:dbl)  [unwired: 4 in]
              "Primary" <- w321
              "Secondary" <- w320
              n93 = call "GEN_ResetTimer.vi"("error in (no error)"=w335, "Data_In"=w325, "Cluster IN"=w329) -> ("error out"=w316:errorcluster, "Data_In 2"=w317:T4, "Cluster OUT"=w318:T6, "TimeStamp"=w310:timestamp)  [unwired: 5 in]
              "Time Stamp" <- w310
              n94 = Enqueue Element(queue=w331, element=cluster{T3, bool} {enum."UpdatePlots", FALSE}) -> ()  [unwired: 2 in, 3 out]
              n95 = call "LCR_GetGlobals.vi"("error in (no error)"=w316, "Data_In"=w317, "Cluster IN"=w318, "Start Stamp"=w310) -> ("error out"=w313:errorcluster, "Data_Out"=w314:T4, "Cluster OUT"=w315:T6, "T Var"=w312:dbl, "T Delta t"=→"T Lag":dbl, "B Var"=w311:dbl, "B Delta t"=→"B Lag":dbl)  [unwired: 1 in]
              "Temperature" <- w312
              "Magnetic Field" <- w311
              n96 = Bundle("Primary Measurement"=w321, "Secondary Measurement"=w320, "T Var"=w312, "B Var"=w311) -> (w319:T11)  [unwired: 1 in]
              n97 = call "LCR_InsertMeasurements.vi"("Data Cluster"=w319, "TimeStamp"=w310, "error in (no error)"=w313, "Data_IN"=w314, "Cluster IN"=w315) -> ("error out"=w327:errorcluster, "Data_OUT"=w323:T4, "Cluster OUT"=w328:T6)  [unwired: 4 in]
              n98 = call "LCR_Logfile.vi"("Data Cluster"=w319, "Time Stamp"=w310, "error in"=w327, "Data_In"=w323, "Config_In"=w328, "FilePrefix"="Logfile Prefix") -> ("error out"=w333:errorcluster, "Data_Out"=w322:T4, "Config_Out"=w332:T6)  [unwired: 3 in]
            }
            frame "ChangeOperation" {
              n99 = property on="Operation Mode" class="RadioBtnsControl (strict)"() -> ("Value"=w349:enum32{"Item 0", "Item 1", "Radio Selection 3"})  [unwired: 2 in, 2 out]
              n100 = case shown="\"Radio Selection 3\"" w349 {
                tunnel: [Mode_Enum."Idle-Off" ("Operation.Operation Mode") Mode_Enum."Idle" ("Operation.Operation Mode") Mode_Enum."Logging" ("Operation.Operation Mode")] -> w345
                frame "Item 0", Default {
                }
                frame "Item 1" {
                }
                frame "Radio Selection 3" {
                }
              }
              n101 = Bundle By Name(cluster=w350, "Operation.Operation Mode"=w345) -> (w347:T6)
              n102 = case shown="\"Logging\", Default" w345 {
                tunnel: ["Measure and logging\n" "Off\n" "Measure only\n"] -> w344
                frame "Logging", Default {
                }
                frame "Idle-Off" {
                }
                frame "Idle" {
                }
              }
              n103 = control-ref of="Status"() -> (w339:refnum<vi>)
              n104 = Concatenate Strings("Changed Mode to: " ("string"), w344) -> (w342:string)
              n105 = call "GEN_WriteStatus.vi"("Input String"=w342, "error in (no error)"=w341, "Config_Cluster"=w347, "Status Ref"=w339) -> ("error out"=w340:errorcluster, "Config_Cluster Out"=w346:T6)  [unwired: 6 in]
            }
            frame "RefreshMUnits" {
              n106 = control-ref of="Primary"() -> (w362:refnum<vi>)
              n107 = control-ref of="Secondary"() -> (w361:refnum<vi>)
              n108 = call "LCR_ReadMType.vi"("error in (no error)"=w365, "Configuration Cluster"=w369) -> ("error out"=w360:errorcluster, "Configuration Cluster Out"=w366:T6, "Secondary Unit"=w363:T12, "Primary Unit"=w364:T12)  [unwired: 6 in]
              n109 = call "LCR_AutoChangeUnits.vi"("Secondary Ref"=w361, "Secondary Unit"=w363, "Primary Ref"=w362, "Primary Unit"=w364) -> ()  [unwired: 8 in]
            }
            frame "UpdatePlots" {
              n110 = control-ref of="Test Graph"() -> (w377:refnum<vi>)
              n111 = call "LCR_PlotHelper.vi"("Y-Axis"="Y-Axis", "X-Axis"="X-Axis", "Data_IN"=w374, "Graph REF"=w377) -> ("Graph Out"=→"Test Graph":cluster{"Variant X":dbl, "Variant Y":dbl}[], "Data_Out"=w373:T4)  [unwired: 6 in]
            }
          }
          n112 = Merge Errors(w28, w29) -> (w39:errorcluster)
          n113 = call "GEN_CulArray.vi"("Max Values"="Max Elements", "Data_Cluster"=w26) -> ("Data_Cluster Out"=w25:T4)  [unwired: 9 in]
          n114 = Or(x=w39, y=w38) -> (x .or. y?=w37:bool)
        }
      }
      frame Error {
      }
    }
  }
  n115 = while {
    tunnel: w3 -> [w384]
    tunnel: w4 -> [w383]
    tunnel: w1 -> [w381]
    stop <- w382 stop-if-true
    # "GUI Event Loop"
    n116 = event shown="[1] \"Exit_Button\": Value Change" {
      selector: _ -> [_ _ _ _ _ _ _ _ _]
      dyn-events: _ -> [_ _ _ _ _ _ _ _ _]
      timeout: _ -> [_ _ _ _ _ _ _ _ _]
      tunnel: w384 -> [_ w389 w394 w399 w404 w409 w414 w419 w424]
      tunnel: w383 -> [_ w388 w393 w398 w403 w408 w413 w418 w423]
      tunnel: [_ TRUE FALSE FALSE FALSE FALSE FALSE FALSE FALSE] -> w382
      tunnel: w381 -> [_ w385 w390 w395 w400 w405 w410 w415 w420]
      event Timeout {
        n117 = event-data() -> ()  [unwired: 1 in, 3 out]
      }
      event "Exit_Button": Value Change {
        n118 = event-data() -> ()  [unwired: 1 in, 6 out]
        n119 = Set Occurrence(w385) -> ()
        n120 = Enqueue Element At Opposite End(queue=w389, element=cluster{T3, bool} {enum."Idle", TRUE}, error in (no error)=w388) -> ()  [unwired: 1 in, 3 out]
      }
      event "Retry_Button": Value Change {
        n121 = event-data() -> ()  [unwired: 1 in, 6 out]
        n122 = Set Occurrence(w390) -> ()
        n123 = Enqueue Element At Opposite End(queue=w394, element=cluster{T3, bool} {enum."RetryComs", FALSE}, error in (no error)=w393) -> ()  [unwired: 1 in, 3 out]
      }
      event "LoadProfile_Button": Value Change {
        n124 = event-data() -> ()  [unwired: 1 in, 6 out]
        n125 = Set Occurrence(w395) -> ()
        n126 = Enqueue Element At Opposite End(queue=w399, element=cluster{T3, bool} {enum."LoadProfile", FALSE}, error in (no error)=w398) -> ()  [unwired: 1 in, 3 out]
      }
      event "SaveProfile_Button": Value Change {
        n127 = event-data() -> ()  [unwired: 1 in, 6 out]
        n128 = Set Occurrence(w400) -> ()
        n129 = Enqueue Element At Opposite End(queue=w404, element=cluster{T3, bool} {enum."SaveProfile", FALSE}, error in (no error)=w403) -> ()  [unwired: 1 in, 3 out]
      }
      event "SaveConfig_Button": Value Change {
        n130 = event-data() -> ()  [unwired: 1 in, 6 out]
        n131 = Set Occurrence(w405) -> ()
        n132 = Enqueue Element At Opposite End(queue=w409, element=cluster{T3, bool} {enum."SaveConfig", FALSE}, error in (no error)=w408) -> ()  [unwired: 1 in, 3 out]
      }
      event "Send_Button": Value Change {
        n133 = event-data() -> ()  [unwired: 1 in, 6 out]
        n134 = Set Occurrence(w410) -> ()
        n135 = Enqueue Element At Opposite End(queue=w414, element=cluster{T3, bool} {enum."SendProfile", FALSE}, error in (no error)=w413) -> ()  [unwired: 1 in, 3 out]
      }
      event "Operation Mode": Value Change {
        n136 = event-data() -> ()  [unwired: 1 in, 6 out]
        n137 = Set Occurrence(w415) -> ()
        n138 = Enqueue Element At Opposite End(queue=w419, element=cluster{T3, bool} {enum."ChangeOperation", FALSE}, error in (no error)=w418) -> ()  [unwired: 1 in, 3 out]
      }
      event "RefreshM_Button": Value Change {
        n139 = event-data() -> ()  [unwired: 1 in, 6 out]
        n140 = Set Occurrence(w420) -> ()
        n141 = Enqueue Element At Opposite End(queue=w424, element=cluster{T3, bool} {enum."RefreshMUnits", FALSE}, error in (no error)=w423) -> ()  [unwired: 1 in, 3 out]
      }
    }
  }
